vi "ReadWrite.Construct.vi"(8 "error in (no error)":errorcluster, 9 "Refs":T1[](array[typedef]) format="%.0x", 10 "Parent":T1 format="%.0x", 11 "ReadWrite in":refnum<class "ReadWrite.lvclass">) -> (0 "error out":errorcluster, 3 "ReadWrite out":refnum<class "ReadWrite.lvclass">)   [LabVIEW 2015, in "Data Access API.lvlib" / "ReadWrite.lvclass"]
uses:
  ReadWrite.lvclass
  <vilib>/NI Veristand/Custom Device API/Custom Device Item Ref.ctl
  <vilib>/NI Veristand/Custom Device API/Data Access Type.ctl
  ReadWrite.lvclass/ReadWrite.ctl
  <vilib>/NI Veristand/Custom Device API/Custom Device API.lvlib
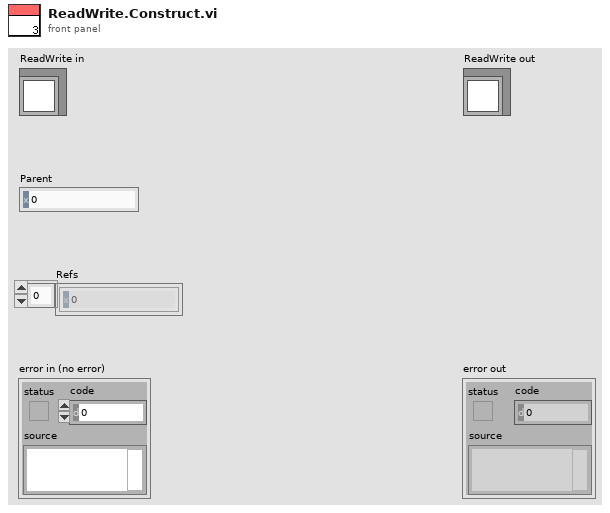
[diagram p1: front panel]
types:
  T1 = typedef "Custom Device API.lvlib/Custom Device Item Ref.ctl" = u64
  T2 = typedef "Custom Device API.lvlib/Data Access Type.ctl" = enum16{"Read", "Write"}
  T3 = typedef "Custom Device API.lvlib/Custom Device Channel.ctl" = cluster{"Type":T4, "Units":string, "Default Value":dbl, "Faultable":bool, "Scalable":bool}
  T4 = typedef "Custom Device API.lvlib/Custom Device Channel Type.ctl" = enum16{"Input", "Output"}
  T5 = typedef "Custom Device API.lvlib/Data Reference.ctl" = i32
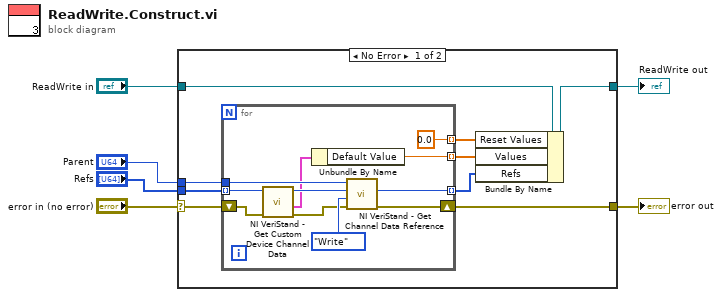
[diagram p0: block diagram]
diagram:
  n1 = case shown="No Error" "error in (no error)" {
    selector: "error in (no error)" -> [w15 w28]
    tunnel: [w14 w28] -> w5
    tunnel: [w12 w27] -> w3
    tunnel: "ReadWrite in" -> [w13 w27]
    tunnel: "Refs" -> [w9 _]
    tunnel: "Parent" -> [w8 _]
    frame No Error {
      n2 = for {
        tunnel: w8 -> [w25]
        tunnel: w9 -> [w23] mode=indexing
        shift-right: [w24] -> w14
        shift-left: w15 -> [w21]
        tunnel: [w18] -> w11 mode=indexing
        tunnel: [w17] -> w10 mode=indexing
        tunnel: [0.0] -> w7 mode=indexing
        n3 = call <vilib>:"NI VeriStand - Get Custom Device Channel Data.vi"("error in (no error)"=w21, "Channel Ref in"=w23) -> ("error out"=w20:errorcluster, "Channel"=w19:T3, "Channel Ref out"=w22:T1)  [unwired: 4 in, 3 out]
        n4 = Unbundle By Name(w19) -> ("Default Value"=w18:dbl)
        n5 = call <vilib>:"NI VeriStand - Get Channel Data Reference.vi"("error in (no error)"=w20, "Access"=Data_Access_Type."Write", "Channel Ref in"=w22, "Device Ref in"=w25) -> ("error out"=w24:errorcluster, "Channel Data Reference"=w17:T5)  [unwired: 5 in, 1 out]
      }
      n6 = Bundle By Name(cluster=w13, "Reset Values"=w7, "Values"=w11, "Refs"=w10) -> (w12:refnum<class "ReadWrite.lvclass">)
    }
    frame Error {
    }
  }
  "error out" <- w5
  "ReadWrite out" <- w3
